vi "Read Strings And Values [].vi"(9 "Ring in":refnum<class "Ring.lvclass">) -> (3 "Ring out":refnum<class "Ring.lvclass">, 4 "Strings And Values []":cluster{"String":string, "Value":variant}[](array[cluster]))   [LabVIEW 2014, in "Raspberry Pi Compatible Compiler for LabVIEW.lvlib" / "Ring.lvclass"]
uses:
  Ring.lvclass
  Ring.lvclass/Ring.ctl
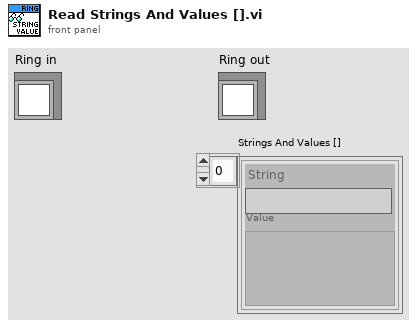
[diagram p1: front panel]
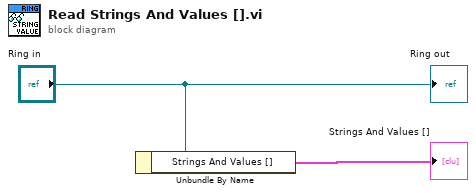
[diagram p0: block diagram]
diagram:
  n1 = Unbundle By Name("Ring in") -> ("Strings And Values []"=→"Strings And Values []":cluster{"String":string, "Value":variant}[])
  "Ring out" <- "Ring in"
